vi "Test NIErrLog Log Provider.vi"   [LabVIEW 2019, in "LVCOOOP Tests.lvlib"]
uses:
  LVCOOOP Tests.lvlib
  LVCOOOP/Utility API/Log Service/public/level.ctl
  9ed7c4c1-ed46-4479-8e22-2070f354f58e.vi
  c2d78877-024c-4e11-b9dd-4a7b3500b578.vi
  3b0b71c3-60f4-4324-8548-373da75483e9.vi
  c9e8b947-a47d-4979-b9d5-80e6d673e01e.vi
  2f095b9b-7ef8-4a73-b6c2-c176aab75462.vi
  d168fba4-da92-4c9c-99b0-20aa9eb51c4f.vi
  e4b81f51-c6e8-4316-94ac-193b1188f7ff.vi
  8c605f87-98e4-45bf-a439-68526c866575.vi
  dbcc2a9b-455d-42eb-bb0c-564023a1863b.vi
  3b0c977e-feed-4995-9e8a-8f6c68ab5002.vi
  c8cf0598-aecd-4ba8-b3e1-8d103b1d9a25.vi
  LVCOOOP/Util/Timestamp or now.vi
  LVCOOOP/Utility API/NIErrLog Log Provider/NIErrLog Log Provider.lvclass
  LVCOOOP/Utility API/Log Service/Log Service.lvclass
panel:
  # "Write messages to the NI Error Log\n\nOn Windows, view the Application Event System Log. Filter on Source = National Instruments Software"
types:
  T1 = typedef "Utility API.lvlib/Log Service.lvclass/level.ctl" = u16
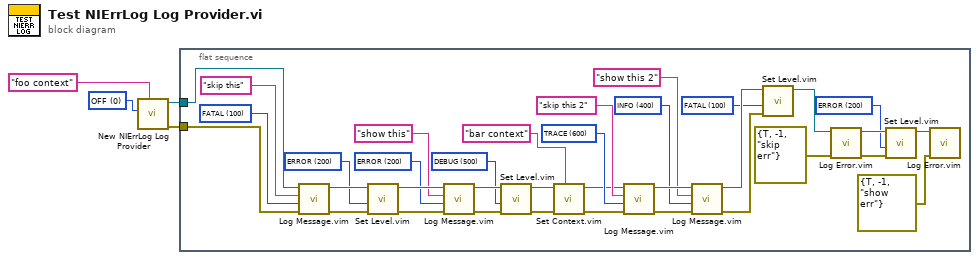
[diagram p0: block diagram]
diagram:
  w3 = T1 0 items=["OFF"=0, "FATAL"=100, "ERROR"=200, "WARN"=300, "INFO"=400, "DEBUG"=500, "TRACE"=600, "ALL"=65535] ("level")
  n1 = call "New NIErrLog Log Provider.vi"("context"="foo context", "level"=w3) -> ("error out"=w1:errorcluster, "Queue Log Provider"=w2:refnum<data-value>)  [unwired: 8 in]
  n2 = flat-sequence {
    tunnel: w2 -> [w39]
    tunnel: w1 -> [w31]
    frame #0 {
      w11 = T1 200 items=["OFF"=0, "FATAL"=100, "ERROR"=200, "WARN"=300, "INFO"=400, "DEBUG"=500, "TRACE"=600, "ALL"=65535] ("level")
      w16 = T1 100 items=["OFF"=0, "FATAL"=100, "ERROR"=200, "WARN"=300, "INFO"=400, "DEBUG"=500, "TRACE"=600, "ALL"=65535] ("level")
      w19 = T1 400 items=["OFF"=0, "FATAL"=100, "ERROR"=200, "WARN"=300, "INFO"=400, "DEBUG"=500, "TRACE"=600, "ALL"=65535] ("level")
      w23 = T1 600 items=["OFF"=0, "FATAL"=100, "ERROR"=200, "WARN"=300, "INFO"=400, "DEBUG"=500, "TRACE"=600, "ALL"=65535] ("level")
      w26 = T1 500 items=["OFF"=0, "FATAL"=100, "ERROR"=200, "WARN"=300, "INFO"=400, "DEBUG"=500, "TRACE"=600, "ALL"=65535] ("level")
      w32 = T1 200 items=["OFF"=0, "FATAL"=100, "ERROR"=200, "WARN"=300, "INFO"=400, "DEBUG"=500, "TRACE"=600, "ALL"=65535] ("level")
      w35 = T1 200 items=["OFF"=0, "FATAL"=100, "ERROR"=200, "WARN"=300, "INFO"=400, "DEBUG"=500, "TRACE"=600, "ALL"=65535] ("level")
      w38 = T1 100 items=["OFF"=0, "FATAL"=100, "ERROR"=200, "WARN"=300, "INFO"=400, "DEBUG"=500, "TRACE"=600, "ALL"=65535] ("level")
      n3 = call "Log Message.vim"("error in (no error)"=w31, "level"=w38, "message"="skip this", "Log Service in"=w39) -> ("error out"=w30:errorcluster, "Log Service out"=w36:refnum<data-value>)  [unwired: 6 in]
      n4 = call "Set Level.vim"("error in (no error)"=w30, "level"=w35, "Log Service in"=w36) -> ("error out"=w29:errorcluster, "Log Service out"=w34:refnum<data-value>)  [unwired: 7 in]
      n5 = call "Log Message.vim"("error in (no error)"=w29, "level"=w32, "message"="show this", "Log Service in"=w34) -> ("error out"=w27:errorcluster, "Log Service out"=w28:refnum<data-value>)  [unwired: 6 in]
      n6 = call "Set Level.vim"("error in (no error)"=w27, "level"=w26, "Log Service in"=w28) -> ("error out"=w7:errorcluster, "Log Service out"=w25:refnum<data-value>)  [unwired: 7 in]
      n7 = call "Set Context.vim"("context"="bar context", "error in (no error)"=w7, "Log Service in"=w25) -> ("error out"=w6:errorcluster, "Log Service out"=w8:refnum<data-value>)  [unwired: 7 in]
      n8 = call "Log Message.vim"("error in (no error)"=w6, "level"=w23, "message"="skip this 2", "Log Service in"=w8) -> ("error out"=w21:errorcluster, "Log Service out"=w22:refnum<data-value>)  [unwired: 6 in]
      n9 = call "Log Message.vim"("error in (no error)"=w21, "level"=w19, "message"="show this 2", "Log Service in"=w22) -> ("error out"=w18:errorcluster, "Log Service out"=w17:refnum<data-value>)  [unwired: 6 in]
      n10 = call "Set Level.vim"("error in (no error)"=w18, "level"=w16, "Log Service in"=w17) -> ("Log Service out"=w15:refnum<data-value>)  [unwired: 7 in, 1 out]
      n11 = call "Log Error.vim"("error in (no error)"=errorcluster {"status"=TRUE, "code"=-1, "source"="skip err"}, "Log Service in"=w15) -> ("error out"=w12:errorcluster, "Log Service out"=w13:refnum<data-value>)  [unwired: 8 in]
      n12 = call "Set Level.vim"("error in (no error)"=w12, "level"=w11, "Log Service in"=w13) -> ("Log Service out"=w10:refnum<data-value>)  [unwired: 7 in, 1 out]
      n13 = call "Log Error.vim"("error in (no error)"=errorcluster {"status"=TRUE, "code"=-1, "source"="show err"}, "Log Service in"=w10) -> ()  [unwired: 8 in, 2 out]
    }
  }
